vi "Write Password file.vi"(8 "error in (no error)":errorcluster, 9 "Access Configuration":T1={"Max ID attempts"=3, "Max password attempts"=4, "Expiration enabled"=TRUE, "Expire days"=90, "User array"=[{"Active?"=TRUE, "User ID"="CTI", "Password"="CTI", "Name"="Mike", "Security level"=10, "Expired?"=FALSE, "Expire sec"=inf, "Locked?"=FALSE, "New?"=TRUE}], "Min password char"=6} {"User array"."Expire sec" format="%.2f"}, 11 "Path":path=path "C:/ProgramData/SDVIS/passwords.txt") -> (0 "error out":errorcluster)   [LabVIEW 2013]
doc: "This vi writes the input Access Configuration Cluster to an encrypted file."
uses:
  User Access Type defs/All users access configuration cluster.ctl
  User Access Type defs/User access cluster array.ctl
  User Access Type defs/User access cluster.ctl
  User Access Type defs/Security level U8.ctl
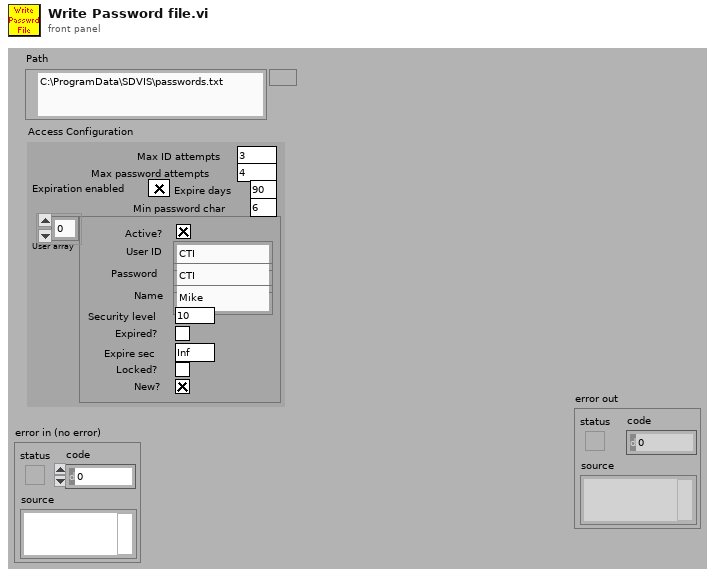
[diagram p1: front panel]
types:
  T1 = typedef "All users access configuration cluster.ctl" = cluster{"Max ID attempts":i32, "Max password attempts":i32, "Expiration enabled":bool, "Expire days":i32, "User array":T2, "Min password char":i32}
  T2 = typedef "User access cluster array.ctl" = T3[]
  T3 = typedef "User access cluster.ctl" = cluster{"Active?":bool, "User ID":string, "Password":string, "Name":string, "Security level":T4, "Expired?":bool, "Expire sec":dbl, "Locked?":bool, "New?":bool}
  T4 = typedef "Security level U8.ctl" = u8
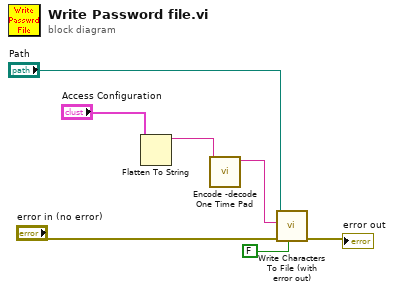
[diagram p0: block diagram]
diagram:
  n1 = Flatten To String(anything="Access Configuration") -> (data string=w1:string)  [unwired: 1 in, 4 out]
  n2 = call "Encode -decode One Time Pad.vi"("Text in"=w1) -> ("Text out"=w3:string)  [unwired: 2 in, 6 out]
  n3 = call "Write Characters To File (with error out).vi"("advisory dialog? (display:T)"=FALSE, "error in (no error)"="error in (no error)", "character string"=w3, "file path (dialog if empty)"="Path") -> ("error out"=→"error out":errorcluster)  [unwired: 3 in, 4 out]
